vi "UPS断电保存全局.vi"() -> ()   [LabVIEW 2016, in "环境动力监测库.lvlib" / "UPS库.lvlib"]
panel:
  in  "型号选择":enum16{"山特UPSC1~3", "山特UPSC6~20"}(ring)
  in  "Serial Config":T1={"baud rate (9600)"=2400, "stop bits (10: 1 bit)"=10, "parity (0:none)"=enum."None", "data bits (8)"=8, "timeout (10sec)"=10000} {"data bits (8)" min=5 max=8 step=1; "stop bits (10: 1 bit)" items=["1.0"=10, "1.5"=15, "2.0"=20]}
  in  "VISA resource name":refnum<visa-resource-name> caption="VISA资源名称"
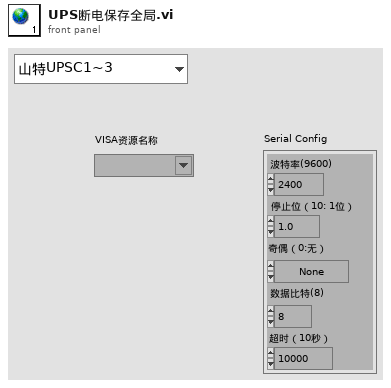
[diagram p1: front panel]
types:
  T1 = cluster{"baud rate (9600)":u32, "stop bits (10: 1 bit)":u16, "parity (0:none)":enum16{"None", "Odd", "Even", "Mark", "Space"}, "data bits (8)":u16, "timeout (10sec)":u32}
diagram:
